vi "String.vi"(1 "#2":dbl, 2 "#1":dbl) -> (0 "Combinada":string)   [LabVIEW 2021]
panel:
  out "Numero Out7":dbl
  out "offset past match":i32
  out "after substring":string
  out "match substring":string
  out "before substring":string
  in  "String":string
  out "#elementos":dbl
  in  "Fim":string
  in  "Início":string
  # "Montar String"
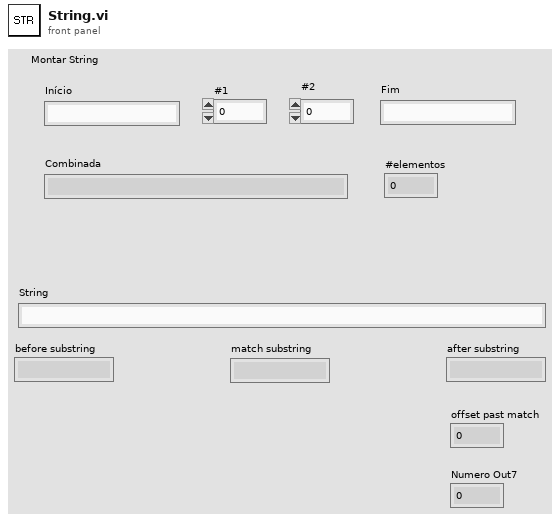
[diagram p1: front panel]
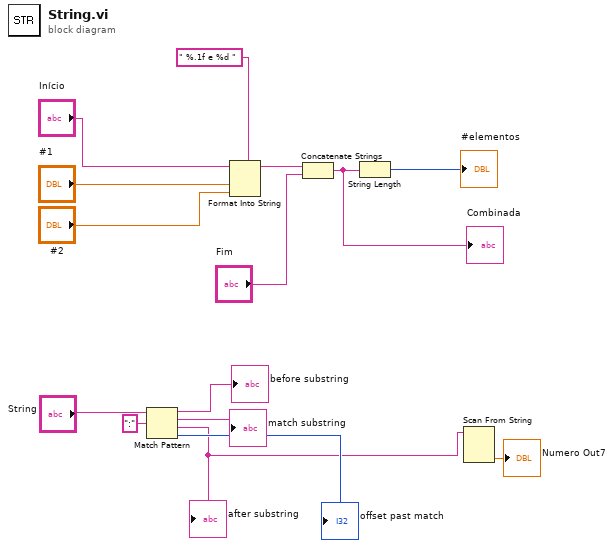
[diagram p0: block diagram]
diagram:
  n1 = Match Pattern(string="String", regular expression=":") -> (before substring=→"before substring":string, match substring=→"match substring":string, after substring=w2:string, offset past match=→"offset past match":i32)  [unwired: 1 in]
  "after substring" <- w2
  n2 = Format Into String(format string=" %.1f e %d ", initial string="Início", "#1", "#2") -> (resulting string=w12:string)  [unwired: 1 in, 1 out]
  n3 = Concatenate Strings(w12, "Fim") -> (w9:string)
  "Combinada" <- w9
  n4 = String Length(string=w9) -> (length=→"#elementos":i32)
  n5 = Scan From String(input string=w2) -> (output 1=→"Numero Out7":dbl)  [unwired: 4 in, 3 out]
